vi "Image Spin.vi"() -> ()   [LabVIEW 2023]
doc: "Rotates a picture file image using LabVIEW. This VI converts the image into a 2D pixmap and uses the Rotate Pixmap VI to rotate the image. \n\nThis VI uses a pixmap array stored on the front panel as a sample image. To use your own image file, click the Use Sample Image? button."
uses:
  Rotate.llb/rotate 24bit.vi
  Rotate.llb/rotate 1bit.vi
  Rotate.llb/rotate 8bit.vi
panel:
  in  "Use Sample Image?":bool=TRUE
  in  "Maintain Center Position?":bool
  in  "Angle Step":dbl=5.0 format="%.2f"
  in  "stop":bool
  out "new picture":picture
  in  "path to file":path
  in  "File Type":enum16{"JPG", "BMP", "PNG"}(ring)=enum."BMP"
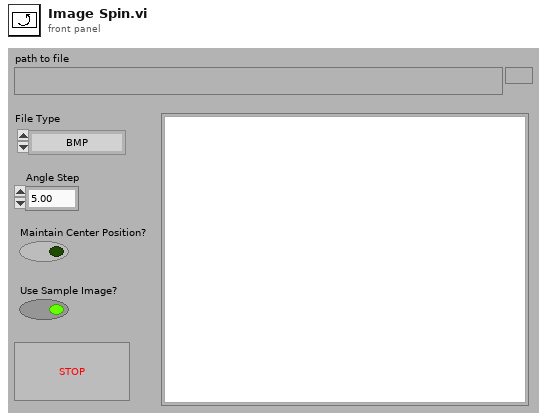
[diagram p1: front panel]
types:
  T1 = cluster{"left":i16, "top":i16, "right":i16, "bottom":i16}
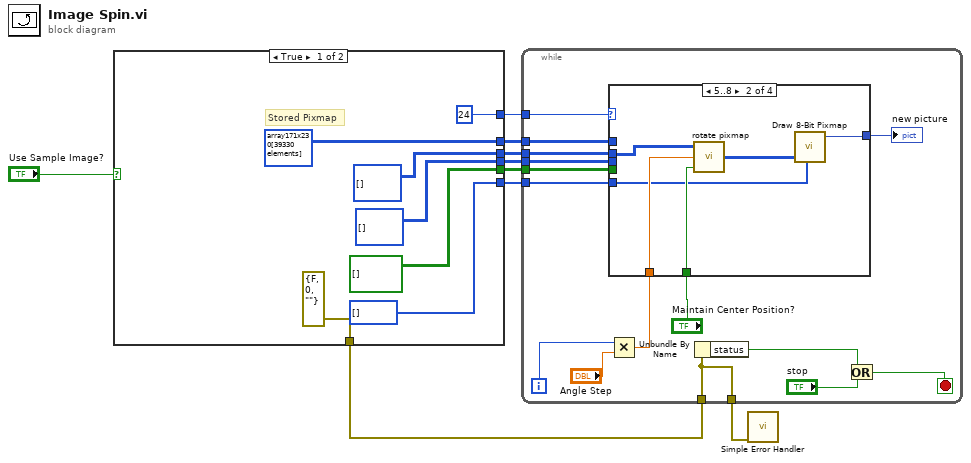
[diagram p0: block diagram]
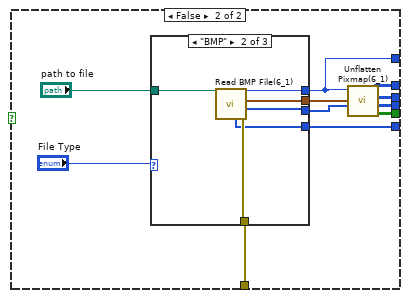
[diagram p2: hidden frame]
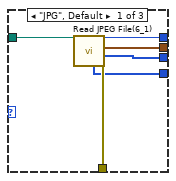
[diagram p3: hidden frame]
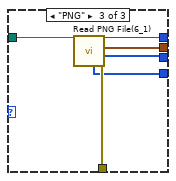
[diagram p4: hidden frame]
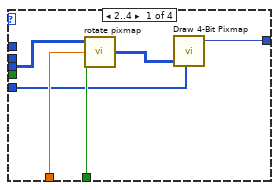
[diagram p5: hidden frame]
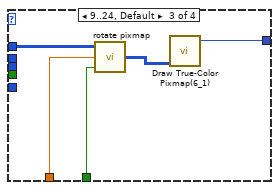
[diagram p6: hidden frame]
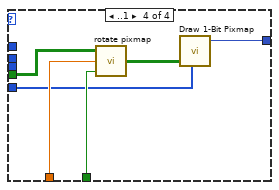
[diagram p7: hidden frame]
diagram:
  n1 = case shown="True" "Use Sample Image?" {
    tunnel: [u32[][] array171x230[39330 elements] ("Array") w23] -> w1
    tunnel: [u8[][] [] ("8-bit pixmap") w22] -> w8
    tunnel: [u8[][] [] ("4-bit pixmap") w21] -> w7
    tunnel: [bool[][] [] ("1-bit pixmap") w20] -> w6
    tunnel: [u32[] [] ("colorTable") w19] -> w5
    tunnel: [24 w18] -> w4
    tunnel: [errorcluster {"status"=FALSE, "code"=0, "source"=""} ("error out") w17] -> w3
    frame True {
      # "Stored Pixmap"
    }
    frame False {
      n2 = case shown="\"BMP\"" "File Type" {
        tunnel: "path to file" -> [w33 w39 w45]
        tunnel: [w32 w38 w44] -> w18
        tunnel: [w31 w37 w43] -> w17
        tunnel: [w30 w36 w42] -> w19
        tunnel: [w29 w35 w41] -> w26
        tunnel: [w28 w34 w40] -> w27
        frame "JPG", Default {
          n3 = call <vilib>:"Read JPEG File(6_1).vi"("path to JPEG file"=w33) -> ("error out"=w31:errorcluster, "flattened image data"=w28:u8[], "rect"=w29:T1, "colorTable"=w30:u32[], "depth"=w32:u8)  [unwired: 5 in, 1 out]
        }
        frame "BMP" {
          n4 = call <vilib>:"Read BMP File(6_1).vi"("path to BMP file"=w39) -> ("error out"=w37:errorcluster, "flattened image data"=w34:u8[], "rect"=w35:T1, "color table"=w36:u32[], "depth"=w38:u8)  [unwired: 5 in, 1 out]
        }
        frame "PNG" {
          n5 = call <vilib>:"Read PNG File(6_1).vi"("path to PNG file"=w45) -> ("error out"=w43:errorcluster, "flattened image data"=w40:u8[], "rect"=w41:T1, "colorTable"=w42:u32[], "depth"=w44:u8)  [unwired: 5 in, 1 out]
        }
      }
      n6 = call <vilib>:"Unflatten Pixmap(6_1).vi"("flattened image data"=w27, "rect"=w26, "depth"=w18) -> ("1-bit pixmap"=w20:bool[][], "4-bit pixmap"=w21:u8[][], "8-bit pixmap"=w22:u8[][], "24-bit pixmap"=w23:u32[][])  [unwired: 4 in, 1 out]
    }
  }
  n7 = while {
    tunnel: w1 -> [w53]
    tunnel: w8 -> [w52]
    tunnel: w7 -> [w51]
    tunnel: w6 -> [w50]
    tunnel: w5 -> [w49]
    tunnel: w4 -> [w48]
    tunnel: w3 -> [w47]
    tunnel: [w47] -> w2
    i -> [w59]
    stop <- w55 stop-if-true
    n8 = Multiply(x=w59, y="Angle Step") -> (x*y=w57:dbl)
    n9 = case shown="5..8" w48 {
      tunnel: w57 -> [w66 w72 w77 w83]
      tunnel: [w64 w70 w75 w82] -> w60
      tunnel: "Maintain Center Position?" -> [w63 w69 w74 w81]
      tunnel: w53 -> [_ _ w73 _]
      tunnel: w52 -> [_ w68 _ _]
      tunnel: w51 -> [w62 _ _ _]
      tunnel: w50 -> [_ _ _ w80]
      tunnel: w49 -> [w61 w67 _ w78]
      frame 2..4 {
        n10 = call-poly "rotate pixmap.vi"("Maintain Center Position?"=w63, "Rotation Angle (degrees)"=w66, "Pixmap"=w62) -> ("Rotated Pixmap"=w65:u8[][])  [unwired: 1 in]
        n11 = call <vilib>:"Draw 4-Bit Pixmap.vi"("data"=w65, "color table"=w61) -> ("new picture"=w64:picture)  [unwired: 7 in]
      }
      frame 5..8 {
        n12 = call-poly "rotate pixmap.vi"("Maintain Center Position?"=w69, "Rotation Angle (degrees)"=w72, "Pixmap"=w68) -> ("Rotated Pixmap"=w71:u8[][])  [unwired: 1 in]
        n13 = call <vilib>:"Draw 8-Bit Pixmap.vi"("data"=w71, "color table"=w67) -> ("new picture"=w70:picture)  [unwired: 7 in]
      }
      frame 9..24, Default {
        n14 = call-poly "rotate pixmap.vi"("Maintain Center Position?"=w74, "Rotation Angle (degrees)"=w77, "Pixmap"=w73) -> ("Rotated Pixmap"=w76:u32[][])  [unwired: 1 in]
        n15 = call <vilib>:"Draw True-Color Pixmap(6_1).vi"("data (RGB format)"=w76) -> ("new picture"=w75:picture)  [unwired: 8 in]
      }
      frame ..1 {
        n16 = call-poly "rotate pixmap.vi"("Maintain Center Position?"=w81, "Rotation Angle (degrees)"=w83, "Pixmap"=w80) -> ("Rotated Pixmap"=w79:bool[][])  [unwired: 1 in]
        n17 = call <vilib>:"Draw 1-Bit Pixmap.vi"("data"=w79, "color table"=w78) -> ("new picture"=w82:picture)  [unwired: 7 in]
      }
    }
    "new picture" <- w60
    n18 = Unbundle By Name(w47) -> ("status"=w46:bool)
    n19 = Or(x=w46, y="stop") -> (x .or. y?=w55:bool)
  }
  n20 = call <vilib>:"Simple Error Handler.vi"("error in (no error)"=w2) -> ()  [unwired: 4 in, 5 out]
